vi "circle perimeter.vi"(2 "spacing between points (1)":u16=1, 3 "arc size (radians)":sgl=6.28319, 4 "arc start (radians)":sgl, 5 "radius":i32) -> (0 "theta":dbl[](array[numeric]), 1 "points along perimeter":cluster{"x":i16, "y":i16}[](array[cluster]))   [LabVIEW 2009]
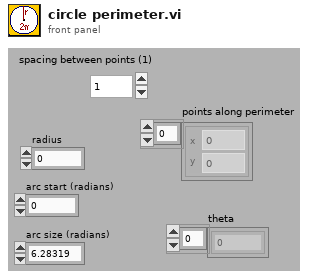
[diagram p1: front panel]
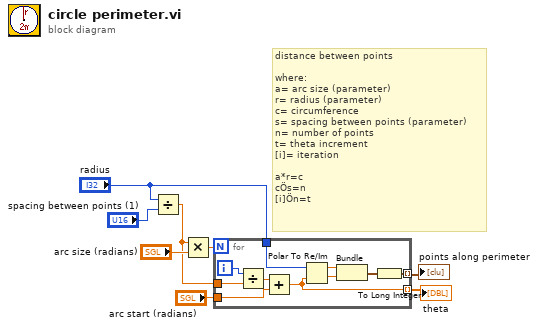
[diagram p0: block diagram]
diagram:
  # "distance between points\n\nwhere:\na= arc size (parameter)\nr= radius (parameter)\nc= circumference\ns= spacing between points (parameter)\nn= number of points\nt= theta increment\n[i]= iteration\n\na*r=c\ncÖs=n\n[i]Ön=t"
  n1 = Divide(x="radius", y="spacing between points (1)") -> (x/y=w2:dbl)
  n2 = Multiply(x=w2, y="arc size (radians)") -> (x*y=w7:dbl)
  n3 = for {
    N: w7 -> [_]
    tunnel: "radius" -> [w18]
    tunnel: [w9] -> w5 mode=indexing
    tunnel: w2 -> [w13]
    tunnel: "arc start (radians)" -> [w11]
    tunnel: [w10] -> w4 mode=indexing
    i -> [w14]
    n4 = Divide(x=w14, y=w13) -> (x/y=w12:dbl)
    n5 = Add(x=w12, y=w11) -> (x+y=w9:dbl)
    n6 = Polar To Re/Im(2:w9, 3:w18) -> (0:w16:dbl, 1:w17:dbl)
    n7 = Bundle(w17, w16) -> (w15:cluster{dbl, dbl})  [unwired: 1 in]
    n8 = To Long Integer(number=w15) -> (32bit integer=w10:cluster{i32, i32})
  }
  "theta" <- w5
  "points along perimeter" <- w4
